vi "Coherent Set wl follow.vi"(8 "error in (no error)":errorcluster, 11 "Wavelength":string) -> (0 "error out":errorcluster, 3 "exit code":u32)   [LabVIEW 2017]
uses:
  Type defs/Coherent commands direct mode.ctl
  Type defs/Commands List.ctl
  Type defs/Coherent comms control.ctl
panel:
  out "Numeric":i32
  out "Time has Elapsed":bool
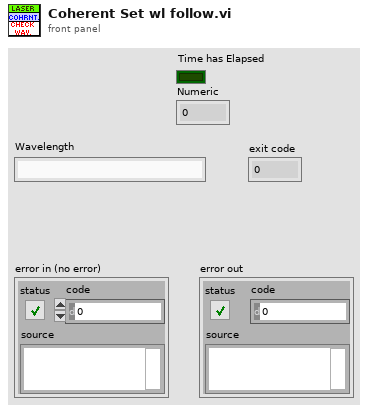
[diagram p1: front panel]
types:
  T1 = typedef "Coherent comms control.ctl" = enum16{"Initialise", "Get Command", "Set Command", "Clear Buffer", "Close"}
  T2 = typedef "Coherent commands direct mode.ctl" = cluster{"Commands & Queries":T3, "Data String":string}
  T3 = typedef "Commands List.ctl" = enum16{"E", "B", "FL", "HM", "L", "LBOH", "LBOOPT", "LFP", "PROMPT", "SM", "S", "VW", "VWS", "HB", "HBR", "REQ", "ALIGN", "K", "F", "FH", "UF", "PHLDC", "PZTMC", "PZTXC", "PZTYC", "PHLDP", "PZTMP", "PZTXP", "PZTYP", "PTRK", "MDLK", "PP", "TS", "STPRPOS", "C", "D1C", "D2C", "BT", "D1T", "D2T", "VT", "LBOT", "ET", "D1ST", "D2ST", "VST", "LBOST", "EST", "D1TD", "D2TD", "VD", "LBOD", "ED", "D1HST", "D2HST", "LRS", "D1SS", "D2SS", "VSS", "LBOSS", "ESS", "D1H", "D2H", "HH", "D1V", "D2V", "SV", "MB", "PI", "BV", "AMDLK", "PZTS", "TMAX", "TMIN", "ALIGNP", "ALIGNW", "PZTXCM", "PZTXCP", "PZTXPM", "PZTXPP", "PZTYCM", "PZTYCP", "PZTYPM", "PZTYPP", "RH", "SN", "ST", "GDDCURVE", "GDD", "GDDCURVEN", "SETCURVEN", "SETCURVEPT", "SAVECURVE", "DELCURVE", "CURVEN", "CURVEPT", "CURVE", "COMP", "HMCOMP", "GDDMAX", "GDDMIN"}
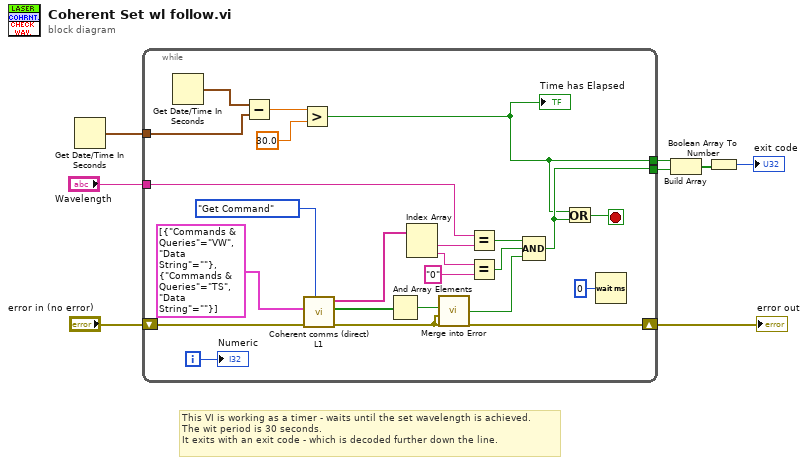
[diagram p0: block diagram]
diagram:
  # "This VI is working as a timer - waits until the set wavelength is achieved.\nThe wit period is 30 seconds.\nIt exits with an exit code - which is decoded further down the line."
  n1 = Get Date/Time In Seconds() -> (seconds since 1Jan1904=w1:timestamp)
  n2 = while {
    shift-right: [w17] -> w8
    shift-left: "error in (no error)" -> [w31]
    tunnel: "Wavelength" -> [w26]
    tunnel: [w10] -> w5
    tunnel: [w19] -> w4
    tunnel: w1 -> [w13]
    i -> [w15]
    stop <- w20 stop-if-true
    n3 = Get Date/Time In Seconds() -> (seconds since 1Jan1904=w14:timestamp)
    n4 = Subtract(x=w14, y=w13) -> (x-y=w12:dbl)
    n5 = Greater?(x=w12, y=30.0) -> (0:w10:bool)
    "Time has Elapsed" <- w10
    n6 = call "Coherent comms (direct) L1.vi"("Coherent laser commands L1"=Coherent_comms_control."Get Command", "error in (no error)"=w31, "Commands \nand Queries"=T2[] [{"Commands & Queries"=enum."VW", "Data String"=""}, {"Commands & Queries"=enum."TS", "Data String"=""}] ("Commands \nand Queries")) -> ("error out"=w17:errorcluster, "Resp Validated ?"=w21:bool[], "Data"=w28:string[])  [unwired: 4 in, 2 out]
    n7 = And Array Elements(Boolean array=w21) -> (logical AND=w18:bool)
    n8 = Index Array(array=w28) -> (element #1=w27:string, element #2=w25:string)  [unwired: 2 in]
    n9 = call "Merge into Error.vi"("Boolean in"=w18, "error in (no error)"=w17) -> ("Boolean out"=w16:bool)  [unwired: 6 in]
    n10 = Equal?(x=w26, y=w27) -> (x = y?=w23:bool)
    n11 = Equal?(x=w25, y="0") -> (x = y?=w22:bool)
    n12 = Compound Arithmetic op=AND(w23, w22, w16) -> (w19:bool)
    n13 = Or(x=w10, y=w19) -> (x .or. y?=w20:bool)
    n14 = Wait (ms)(milliseconds to wait=u32 0) -> ()  [unwired: 1 out]
    "Numeric" <- w15
  }
  "error out" <- w8
  n15 = Build Array(w5, w4) -> (w3:bool[])
  n16 = Boolean Array To Number(Boolean array=w3) -> (number=→"exit code":u32)
